vi "Message Handler.vi"(8 "error in (no error)":errorcluster, 11 "PID Loop in":refnum<class "PID Loop.lvclass">) -> (0 "error out":errorcluster, 3 "OOQMH out":refnum<class "OOQMH.lvclass">)   [LabVIEW 2024, in "PID Loop.lvlib" / "PID Loop.lvclass"]
uses:
  PID Loop.lvclass
  PID Loop.lvclass/PID Loop.ctl
  OOQMH/OOQMH/OOQMH.lvclass
panel:
  out "Waveform Chart 2":u32(graph)
  out "Waveform Chart":dbl(graph)
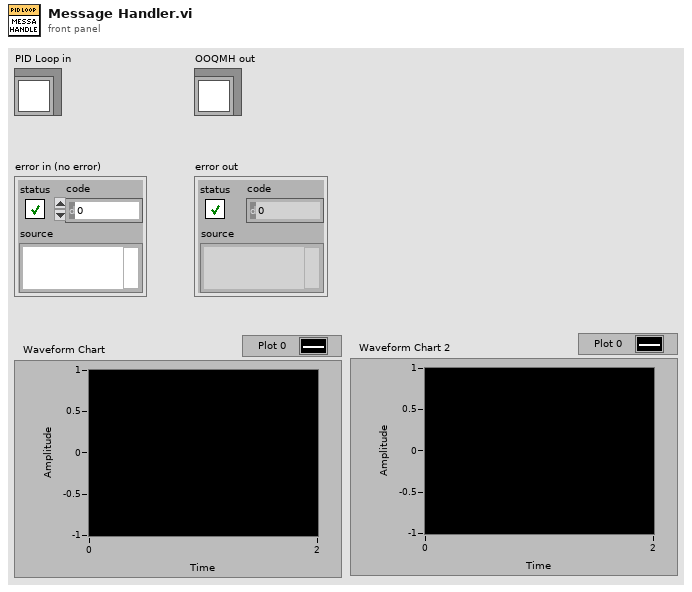
[diagram p1: front panel]
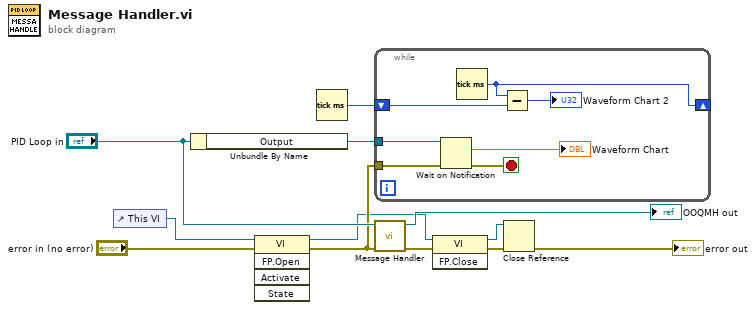
[diagram p0: block diagram]
diagram:
  n1 = control-ref of="This VI"() -> (w9:refnum<vi>)
  n2 = Unbundle By Name("PID Loop in") -> ("Output"=w10:refnum<notifier>)
  n3 = invoke class="VI" method="FP.Open"(reference=w9, error in="error in (no error)") -> (reference out=w2:refnum<vi>, error out=w7:errorcluster)  [unwired: 3 in, 3 out]
  n4 = Tick Count (ms)() -> (millisecond timer value=w1:u32)
  n5 = while {
    tunnel: w10 -> [w19]
    tunnel: w7 -> [w18]
    shift-right: [w14] -> _
    shift-left: w1 -> [w15]
    stop <- w17 stop-if-true
    n6 = Wait on Notification(notifier=w19, error in (no error)=w18) -> (notification=→"Waveform Chart":dbl, error out=w17:errorcluster)  [unwired: 2 in, 2 out]
    n7 = Tick Count (ms)() -> (millisecond timer value=w14:u32)
    n8 = Subtract(x=w14, y=w15) -> (x-y=→"Waveform Chart 2":u32)
  }
  n9 = call-parent "Message Handler.vi"("error in (no error)"=w7, "OOQMH in"="PID Loop in") -> ("error out"=w4:errorcluster, "OOQMH out"=→"OOQMH out":refnum<class "OOQMH.lvclass">)  [unwired: 8 in]
  n10 = invoke class="VI" method="FP.Close"(reference=w2, error in=w4) -> (reference out=w6:refnum<vi>, error out=w5:errorcluster)  [unwired: 1 in, 1 out]
  n11 = Close Reference(reference=w6, error in (no error)=w5) -> (error out=→"error out":errorcluster)
